vi "h.DETECTION.UpdateDetectionSetting.vi"(8 "error in":errorcluster, 10 "Detection Setting":T1, 11 "Connection ID":refnum<k5>) -> (0 "error out":errorcluster, 3 "Connection ID out":refnum<k5>)   [LabVIEW 2016, in "h.Library.lvlib"]
uses:
  h.Library.lvlib
  h.DETECTION.PeakDetectionPreset.ctl
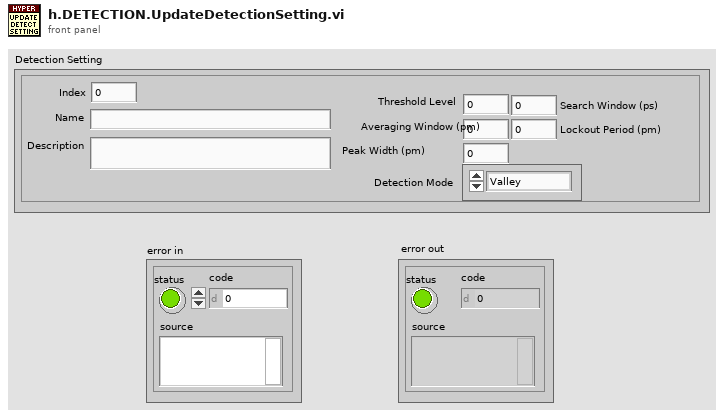
[diagram p1: front panel]
types:
  T1 = typedef "h.Library.lvlib/h.DETECTION.PeakDetectionPreset.ctl" = cluster{"Index":u8, "Name":string, "Description":string, "Detection Mode":enum32{"Valley", "Peak"}, "Averaging Window (pm)":i32, "Peak Width (pm)":i32, "Lockout Period (pm)":i32, "Search Window (ps)":i32, "Threshold Level":i32}
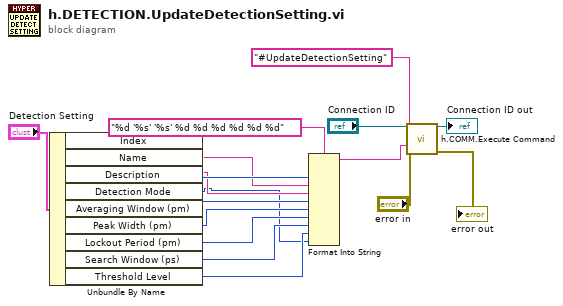
[diagram p0: block diagram]
diagram:
  n1 = Unbundle By Name("Detection Setting") -> ("Index"=w15:u8, "Name"=w14:string, "Description"=w13:string, "Detection Mode"=w7:enum32{"Valley", "Peak"}, "Averaging Window (pm)"=w12:i32, "Peak Width (pm)"=w11:i32, "Lockout Period (pm)"=w10:i32, "Search Window (ps)"=w9:i32, "Threshold Level"=w8:i32)
  n2 = Format Into String(format string="%d '%s' '%s' %d %d %d %d %d %d", w15, w14, w13, w12, w11, w10, w9, w8, w7) -> (resulting string=w1:string)  [unwired: 2 in, 1 out]
  n3 = call "h.COMM.Execute Command.vi"("Connection ID"="Connection ID", "Command"="#UpdateDetectionSetting", "Argument"=w1, "error in"="error in") -> ("Connection ID out"=→"Connection ID out":refnum<k5>, "error out"=→"error out":errorcluster)  [unwired: 4 in, 6 out]
